vi "GEOM_ReadDetInfo.vi"(8 "error in (no error)":errorcluster, 11 "file path":path) -> (0 "error out":errorcluster, 2 "Info":string[][](table), 3 "file path out":path)   [LabVIEW 2016]
uses:
  <vilib>/Utility/config.llb/Read Key (String).vi
  <vilib>/Utility/config.llb/NI_LVConfig.lvlib
panel:
  in  "section":string="INFO"
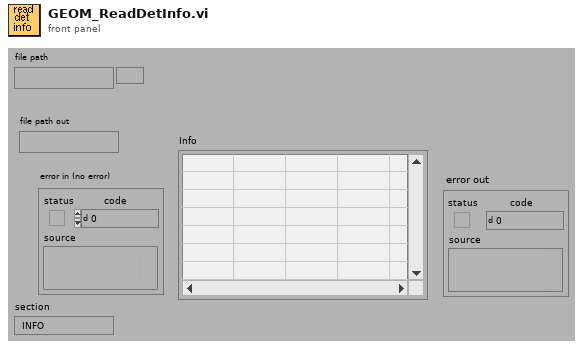
[diagram p1: front panel]
types:
  T1 = typedef "NI_LVConfig.lvlib/Config Data RefNum.ctl" = refnum<k1>
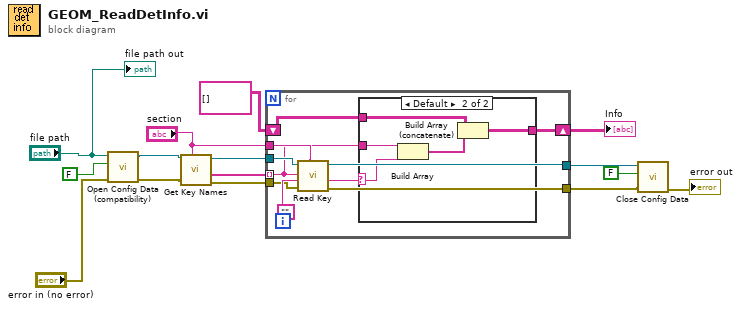
[diagram p0: block diagram]
diagram:
  n1 = call <vilib>:"Open Config Data (compatibility).vi"("error in (no error)"="error in (no error)", "create file if necessary (T)"=FALSE ("create file if necessary? (T)"), "configuration file path"="file path") -> ("error out"=w13:errorcluster, "refnum"=w14:T1)  [unwired: 6 in, 1 out]
  n2 = call <vilib>:"Get Key Names.vi"("section"="section", "error in (no error)"=w13, "refnum"=w14) -> ("error out"=w8:errorcluster, "key names"=w12:string[], "refnum out"=w11:T1)  [unwired: 6 out]
  n3 = for {
    tunnel: w12 -> [w22] mode=indexing
    tunnel: "section" -> [w25]
    tunnel: w11 -> [w24]
    shift-right: [w21] -> w10
    shift-left: string[][] [] -> [w20]
    tunnel: [w19] -> w9
    tunnel: w8 -> [w18]
    tunnel: [w17] -> w2
    n4 = call-poly <vilib>:"Read Key.vi"("section"=w25, "error in (no error)"=w18, "default value"="", "key"=w22, "refnum"=w24) -> ("error out"=w17:errorcluster, "value"=w16:string, "refnum out"=w19:T1)  [unwired: 1 in, 3 out]
    n5 = case shown="Default" w16 {
      selector: w16 -> [_ w27]
      tunnel: w22 -> [_ w31]
      tunnel: [w26 w29] -> w21
      tunnel: w20 -> [w26 w28]
      frame "", " " {
      }
      frame Default {
        n6 = Build Array(w31, w27) -> (w30:string[])
        n7 = Build Array (concatenate)(w28, w30) -> (w29:string[][])
      }
    }
  }
  "Info" <- w10
  n8 = call <vilib>:"Close Config Data.vi"("error in (no error)"=w2, "write file if changed (T)"=FALSE ("write configuration file? (F)"), "refnum"=w9) -> ("error out"=→"error out":errorcluster)  [unwired: 8 out]
  "file path out" <- "file path"
